vi "Start.vi"(8 "error in (no error)":errorcluster, 11 "Panel State Data In":T2={"FGEN Resource"="", "DAQmx Tasks Session"={"DO Task"="", "Ctr0 Task"=""}, "Scope Resource"="", "FGEN Enabled?"=FALSE, "DAQ Enabled?"=FALSE, "Scope Enabled?"=FALSE, "Max Total FGEN Wfm Duration (s)"=0.0, "FGEN-DAQ Routing"={"FGEN Start Trigger"="", "DAQ Trig Line"=""}, "Scope Recording Settings"={"Number of Records"=0, "Channels Per Record"=1, "Plot Names"=[], "Fetch Timeout"=0.0, "Channel List"=""}} {"Scope Recording Settings"."Fetch Timeout" format="%.2f"}) -> (0 "error out":errorcluster, 2 "Actual Sample Rates":T1 {"FGEN Sample Rate" format="%#_6pHz"; "DAQ Sample Rate" format="%#_6pHz"; "SCOPE Sample Rate" format="%#_6pHz"}, 3 "Panel State Data Out":T2={"FGEN Resource"="", "DAQmx Tasks Session"={"DO Task"="", "Ctr0 Task"=""}, "Scope Resource"="", "FGEN Enabled?"=FALSE, "DAQ Enabled?"=FALSE, "Scope Enabled?"=FALSE, "Max Total FGEN Wfm Duration (s)"=0.0, "FGEN-DAQ Routing"={"FGEN Start Trigger"="", "DAQ Trig Line"=""}, "Scope Recording Settings"={"Number of Records"=0, "Channels Per Record"=1, "Plot Names"=[], "Fetch Timeout"=0.0, "Channel List"=""}} {"Scope Recording Settings"."Fetch Timeout" format="%.2f"})   [LabVIEW 2025]
uses:
  <resource>/objmgr/daqmx.rc
  Typedef/Test Panel State Data.ctl
  Typedef/Scope Recording Settings.ctl
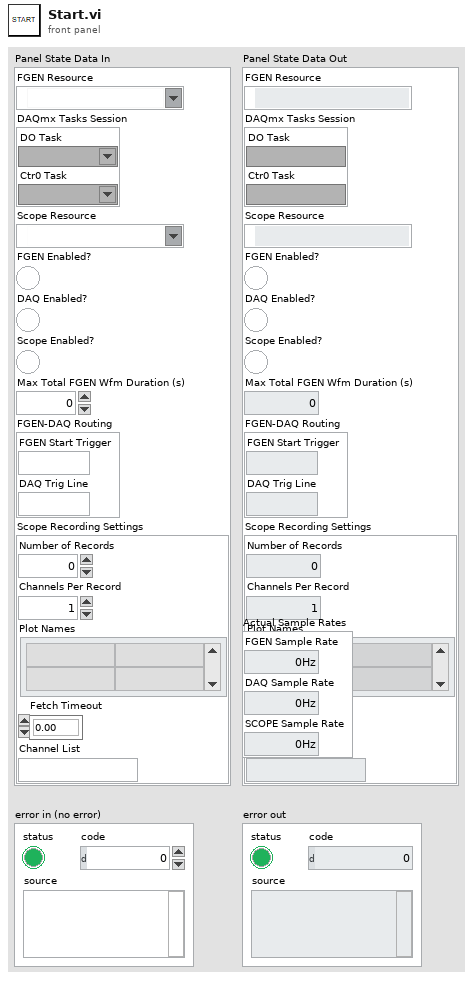
[diagram p1: front panel]
types:
  T1 = cluster{"FGEN Sample Rate":dbl, "DAQ Sample Rate":dbl, "SCOPE Sample Rate":dbl}
  T2 = typedef "Test Panel State Data.ctl" = cluster{"FGEN Resource":refnum<k15>, "DAQmx Tasks Session":cluster{"DO Task":refnum<k21>, "Ctr0 Task":refnum<k21>}, "Scope Resource":refnum<k15>, "FGEN Enabled?":bool, "DAQ Enabled?":bool, "Scope Enabled?":bool, "Max Total FGEN Wfm Duration (s)":dbl, "FGEN-DAQ Routing":cluster{"FGEN Start Trigger":string, "DAQ Trig Line":string}, "Scope Recording Settings":T3}
  T3 = typedef "Scope Recording Settings.ctl" = cluster{"Number of Records":i32, "Channels Per Record":i32, "Plot Names":string[][], "Fetch Timeout":dbl, "Channel List":string}
  T4 = enum16{"Reset", "Start", "Read", "Pause", "Resume"}
  T5 = cluster{"Actual Arb Sample Rate":dbl, "SampClk.Rate":dbl, "Actual Sample Rate":dbl}
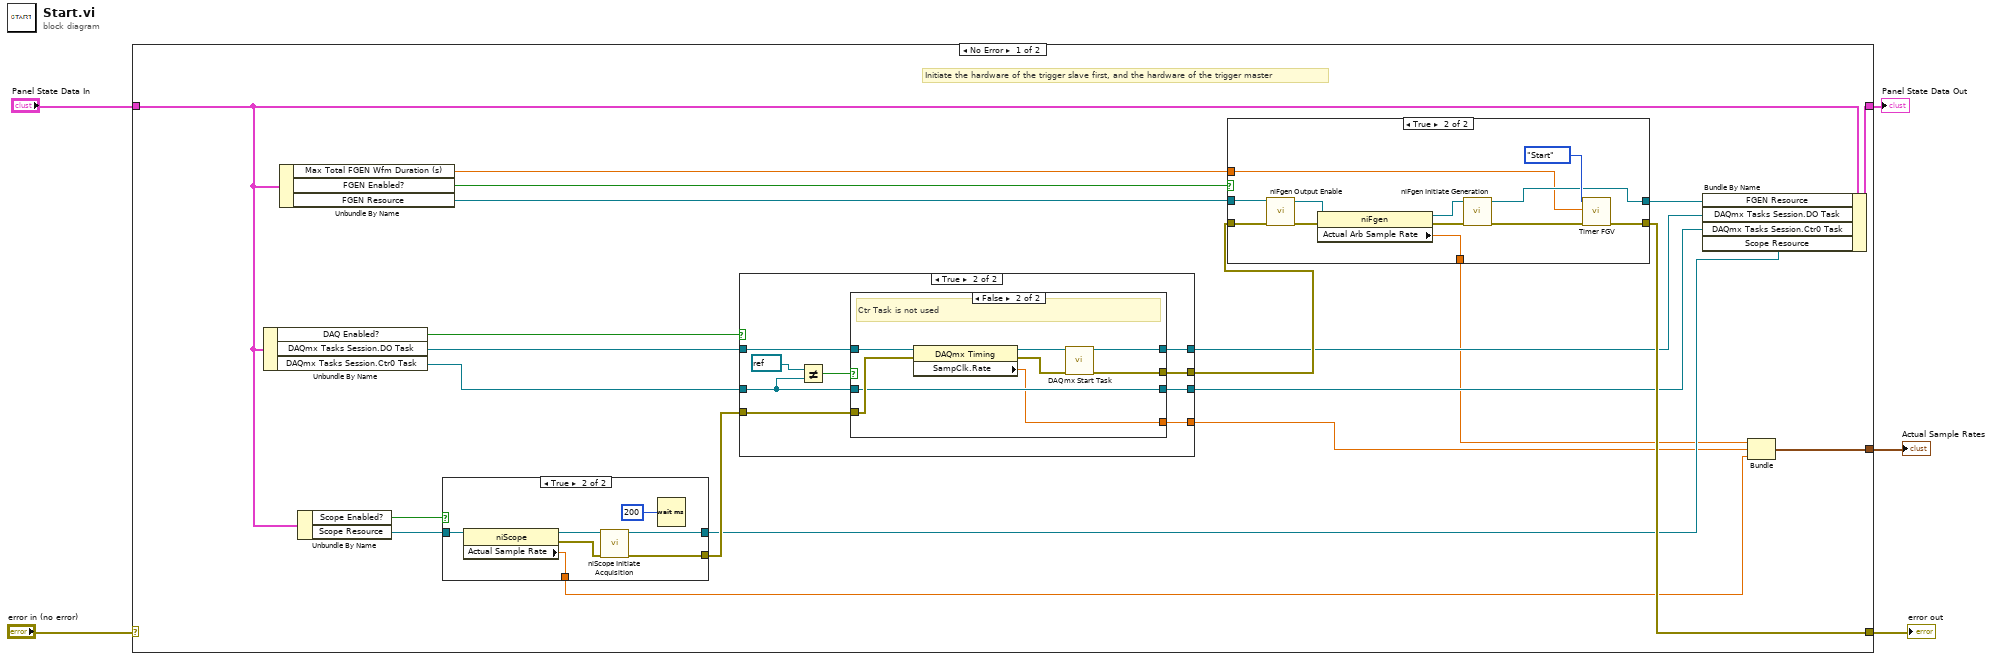
[diagram p0: block diagram]
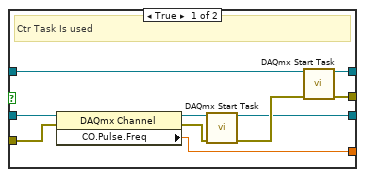
[diagram p4: hidden frame]
diagram:
  n1 = case shown="No Error" "error in (no error)" {
    selector: "error in (no error)" -> [_ w80]
    tunnel: "Panel State Data In" -> [w20 w79]
    tunnel: [w17 w80] -> w5
    tunnel: [w16 w79] -> w2
    tunnel: [w7 _] -> w1
    frame No Error {
      # "Initiate the hardware of the trigger slave first, and the hardware of the trigger master"
      n2 = Unbundle By Name(w20) -> ("DAQ Enabled?"=w23:bool, "DAQmx Tasks Session.DO Task"=w24:refnum<k21>, "DAQmx Tasks Session.Ctr0 Task"=w6:refnum<k21>)
      n3 = Unbundle By Name(w20) -> ("Max Total FGEN Wfm Duration (s)"=w12:dbl, "FGEN Enabled?"=w26:bool, "FGEN Resource"=w25:refnum<k15>)
      n4 = Unbundle By Name(w20) -> ("Scope Enabled?"=w22:bool, "Scope Resource"=w21:refnum<k15>)
      n5 = case shown="True" w22 {
        tunnel: w21 -> [w27 w33]
        tunnel: [_ w34] -> w19
        tunnel: [w27 w32] -> w13
        tunnel: [_ w28] -> w8
        frame False {
        }
        frame True {
          n6 = property class="niScope"(reference=w33) -> (reference out=w30:refnum<k15>, error out=w29:errorcluster, "Actual Sample Rate"=w28:dbl)  [unwired: 1 in]
          n7 = call <instrlib>:"niScope Initiate Acquisition.vi"("instrument handle"=w30, "error in"=w29) -> ("instrument handle out"=w32:refnum<k15>, "error out"=w34:errorcluster)  [unwired: 12 in]
          n8 = Wait (ms)(milliseconds to wait=u32 200) -> ()  [unwired: 1 out]
        }
      }
      n9 = case shown="True" w23 {
        tunnel: w24 -> [w36 w46]
        tunnel: [w37 w45] -> w18
        tunnel: w19 -> [w37 w44]
        tunnel: [w36 w43] -> w14
        tunnel: w6 -> [w35 w40]
        tunnel: [w35 w42] -> w11
        tunnel: [_ w41] -> w9
        frame False {
        }
        frame True {
          n10 = Not Equal?(x=refnum<k21> refnum ("DAQmx Tasks Session.Ctr0 Task"), y=w40) -> (x != y?=w38:bool)
          n11 = case shown="False" w38 {
            tunnel: w46 -> [w56 w59]
            tunnel: [w55 w64] -> w45
            tunnel: w44 -> [w54 w63]
            tunnel: [w53 w62] -> w43
            tunnel: [w51 w61] -> w42
            tunnel: [w48 w57] -> w41
            tunnel: w40 -> [w47 w61]
            frame True {
              # "Ctr Task Is used"
              n12 = property class="DAQmx Channel"(reference=w47, error in=w54) -> (reference out=w49:refnum<k21>, error out=w50:errorcluster, "CO.Pulse.Freq"=w48:dbl)
              n13 = call <vilib>:"DAQmx Start Task.vi"("task/channels in"=w49, "error in"=w50) -> ("task out"=w51:refnum<k21>, "error out"=w52:errorcluster)  [unwired: 12 in]
              n14 = call <vilib>:"DAQmx Start Task.vi"("task/channels in"=w56, "error in"=w52) -> ("task out"=w53:refnum<k21>, "error out"=w55:errorcluster)  [unwired: 12 in]
            }
            frame False {
              # "Ctr Task is not used"
              n15 = property class="DAQmx Timing"(reference=w59, error in=w63) -> (reference out=w58:refnum<k21>, error out=w60:errorcluster, "SampClk.Rate"=w57:dbl)
              n16 = call <vilib>:"DAQmx Start Task.vi"("task/channels in"=w58, "error in"=w60) -> ("task out"=w62:refnum<k21>, "error out"=w64:errorcluster)  [unwired: 12 in]
            }
          }
        }
      }
      n17 = case shown="True" w26 {
        tunnel: w25 -> [w65 w76]
        tunnel: [w66 w73] -> w17
        tunnel: w18 -> [w66 w78]
        tunnel: [w65 w72] -> w15
        tunnel: w12 -> [_ w71]
        tunnel: [_ w67] -> w10
        frame False {
        }
        frame True {
          n18 = call <instrlib>:"niFgen Output Enable.vi"("error in (no error)"=w78, "Instrument Handle"=w76) -> ("error out"=w77:errorcluster, "Instrument Handle Out"=w69:refnum<k15>)  [unwired: 8 in]
          n19 = property class="niFgen"(reference=w69, error in=w77) -> (reference out=w68:refnum<k15>, error out=w70:errorcluster, "Actual Arb Sample Rate"=w67:dbl)
          n20 = call <instrlib>:"niFgen Initiate Generation.vi"("error in (no error)"=w70, "Instrument Handle"=w68) -> ("error out"=w74:errorcluster, "Instrument Handle Out"=w72:refnum<k15>)  [unwired: 8 in]
          n21 = call "Timer FGV.vi"("error in (no error)"=w74, "Time target (s)"=w71, "Timer mode"=T4."Start") -> ("error out"=w73:errorcluster)  [unwired: 5 in, 3 out]
        }
      }
      n22 = Bundle By Name(cluster=w20, "FGEN Resource"=w15, "DAQmx Tasks Session.DO Task"=w14, "DAQmx Tasks Session.Ctr0 Task"=w11, "Scope Resource"=w13) -> (w16:T2)
      n23 = Bundle("Actual Arb Sample Rate"=w10, "SampClk.Rate"=w9, "Actual Sample Rate"=w8) -> (w7:T5)  [unwired: 1 in]
    }
    frame Error {
    }
  }
  "error out" <- w5
  "Panel State Data Out" <- w2
  "Actual Sample Rates" <- w1
